vi "S2C_ManageError.vi"(8 "Error In":errorcluster) -> (0 "Error Out":errorcluster)   [LabVIEW 2015]
doc: "Write an error to file, displays the error to the user, and exits the application if warranted."
uses:
  <vilib>/Utility/error.llb/DialogType.ctl
  Globals/S2C_Globals.vi
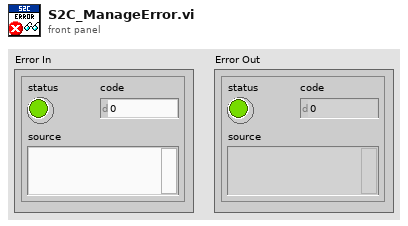
[diagram p1: front panel]
types:
  T1 = typedef "DialogType.ctl" = u16
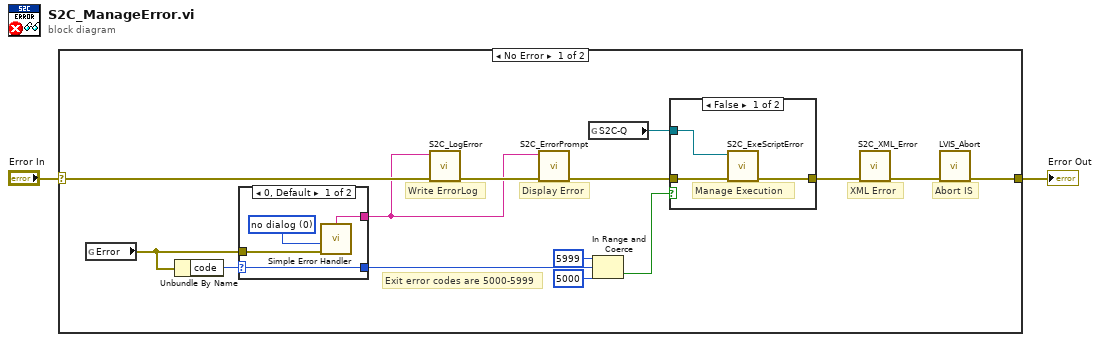
[diagram p0: block diagram]
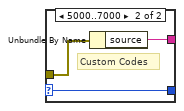
[diagram p2: hidden frame]
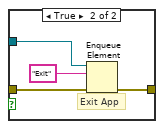
[diagram p3: hidden frame]
diagram:
  n1 = case shown="No Error" "Error In" {
    selector: "Error In" -> [w13 w31]
    tunnel: [w9 w31] -> w1
    frame No Error {
      # "XML Error"
      # "Abort IS"
      # "Exit error codes are 5000-5999"
      # "Display Error"
      # "Write ErrorLog"
      n2 = global read "S2C_Globals.vi" "Error"() -> (w7:errorcluster)
      n3 = Unbundle By Name(w7) -> ("code"=w6:i32)
      n4 = case shown="0, Default" w6 {
        selector: w6 -> [w17 w21]
        tunnel: w7 -> [w20 w23]
        tunnel: [w18 w22] -> w8
        tunnel: [w17 w21] -> w5
        frame 0, Default {
          w19 = T1 0 items=["no dialog", "OK message", "continue or stop message", "OK message + warnings", "continue/stop + warnings"] ("type of dialog (OK msg:1)")
          n5 = call <vilib>:"Simple Error Handler.vi"("type of dialog (OK msg:1)"=w19, "error in (no error)"=w20) -> ("message"=w18:string)  [unwired: 3 in, 4 out]
        }
        frame 5000..7000 {
          # "Custom Codes"
          n6 = Unbundle By Name(w23) -> ("source"=w22:string)
        }
      }
      n7 = call "S2C_LogError.vi"("Error In"=w13, "Error Msg"=w8) -> ("Error Out"=w16:errorcluster)  [unwired: 9 in]
      n8 = call "S2C_ErrorPrompt.vi"("Error In"=w16, "ErrMsgIn"=w8) -> ("Error Out"=w12:errorcluster)  [unwired: 9 in]
      n9 = global read "S2C_Globals.vi" "S2C-Q"() -> (w10:refnum<queue>)
      n10 = In Range and Coerce(upper limit=5999, x=w5, lower limit=5000) -> (In Range?=w11:bool)  [unwired: 1 out]
      n11 = case shown="False" w11 {
        tunnel: w12 -> [w26 w30]
        tunnel: [w25 w29] -> w4
        tunnel: w10 -> [w24 w27]
        frame False {
          # "Manage Execution"
          n12 = call "S2C_ExeScriptError.vi"("Error In"=w26, "Q-Ref"=w24) -> ("Error Out"=w25:errorcluster)  [unwired: 9 in]
        }
        frame True {
          # "Exit App"
          n13 = Enqueue Element(queue=w27, element="Exit", error in (no error)=w30) -> (error out=w29:errorcluster)  [unwired: 1 in, 2 out]
        }
      }
      n14 = call "S2C_XML_Error.vi"("Error In"=w4) -> ("Error Out"=w3:errorcluster)  [unwired: 10 in]
      n15 = call "LVIS_Abort.vi"("Error In"=w3) -> ("Error Out"=w9:errorcluster)  [unwired: 10 in]
    }
    frame Error {
    }
  }
  "Error Out" <- w1
